vi "TemperatureMeasurePT.vi"(1 "FieldPoint IO Point In":refnum<k21>) -> (0 "Ch1 [K]":dbl)   [LabVIEW 2012]
uses:
  <vilib>/FieldPoint/Polymorphic Read.llb/FP Read (Float -IO).vi
panel:
  in  "?":bool
  # "Temperature Measurement (PT 100)"
  # "(Recommended excitation 1 mA)"
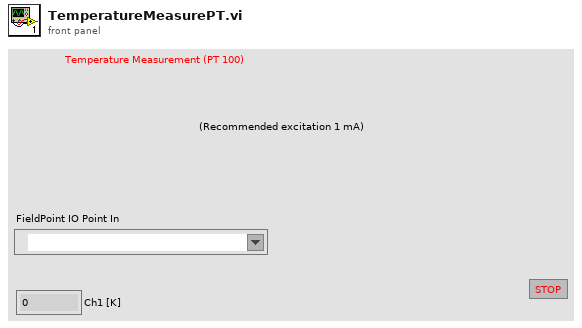
[diagram p1: front panel]
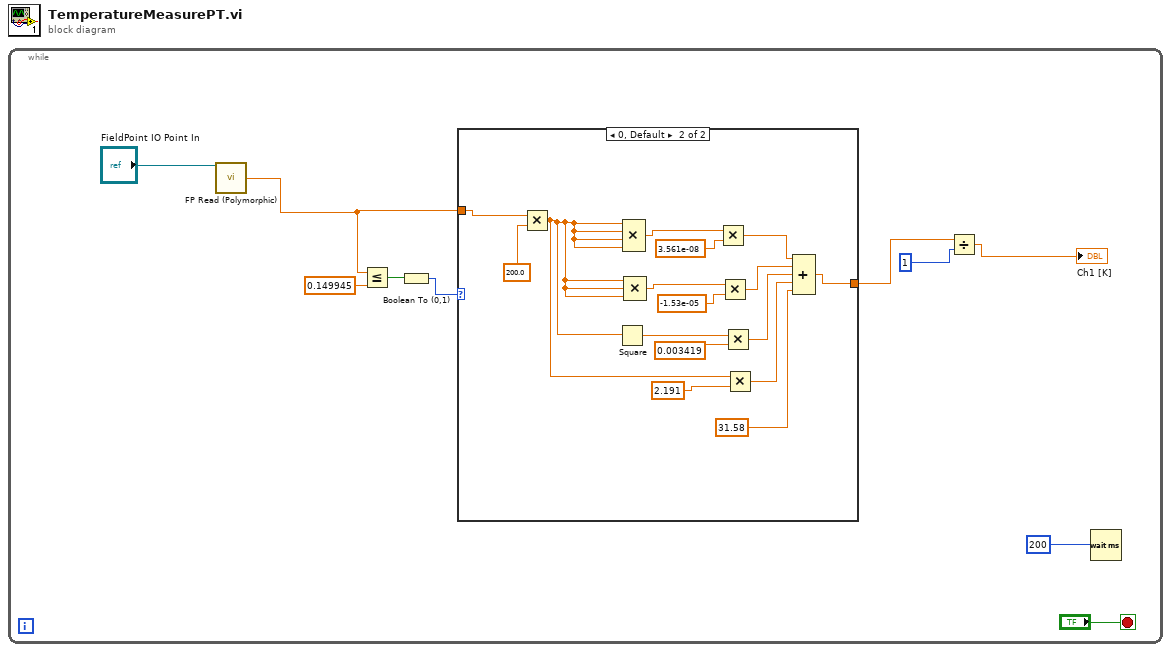
[diagram p0: block diagram]
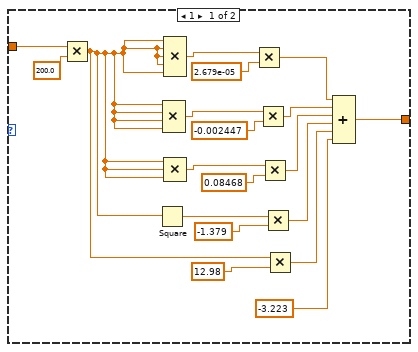
[diagram p2: hidden frame]
diagram:
  n1 = while {
    stop <- "?" stop-if-true
    n2 = call-poly <vilib>:"FP Read (Polymorphic).vi"("FieldPoint IO Point In"="FieldPoint IO Point In") -> ("value"=w4:dbl)  [unwired: 11 in, 3 out]
    n3 = Less Or Equal?(x=w4, y=0.149945) -> (x <= y?=w7:bool)
    n4 = Boolean To (0,1)(Boolean=w7) -> (0, 1=w6:i16)
    n5 = case shown="0, Default" w6 {
      tunnel: w4 -> [w28 w33]
      tunnel: [w17 w31] -> w5
      frame 1 {
        n6 = Multiply(x=w28, y=200.0) -> (x*y=w19:dbl)
        n7 = Square(x=w19) -> (x^2=w21:dbl)
        n8 = Compound Arithmetic op=MULTIPLY(w19, w19, w19, w19) -> (w25:dbl)
        n9 = Compound Arithmetic op=MULTIPLY(w19, w19, w19, w19, w19) -> (w27:dbl)
        n10 = Compound Arithmetic op=MULTIPLY(w19, w19, w19) -> (w23:dbl)
        n11 = Multiply(x=w27, y=2.679e-05) -> (x*y=w16:dbl)
        n12 = Multiply(x=w25, y=-0.002447) -> (x*y=w15:dbl)
        n13 = Multiply(x=w23, y=0.08468) -> (x*y=w14:dbl)
        n14 = Multiply(x=w21, y=-1.379) -> (x*y=w13:dbl)
        n15 = Multiply(x=w19, y=12.98) -> (x*y=w12:dbl)
        n16 = Compound Arithmetic op=ADD(w16, w15, w14, w13, w12, -3.223) -> (w17:dbl)
      }
      frame 0, Default {
        n17 = Multiply(x=w33, y=200.0) -> (x*y=w39:dbl)
        n18 = Square(x=w39) -> (x^2=w41:dbl)
        n19 = Compound Arithmetic op=MULTIPLY(w39, w39, w39, w39) -> (w45:dbl)
        n20 = Compound Arithmetic op=MULTIPLY(w39, w39, w39) -> (w43:dbl)
        n21 = Multiply(x=w45, y=3.561e-08) -> (x*y=w30:dbl)
        n22 = Multiply(x=w43, y=-1.53e-05) -> (x*y=w37:dbl)
        n23 = Multiply(x=w41, y=0.003419) -> (x*y=w36:dbl)
        n24 = Multiply(x=w39, y=2.191) -> (x*y=w35:dbl)
        n25 = Compound Arithmetic op=ADD(w30, w37, w36, w35, 31.58) -> (w31:dbl)
      }
    }
    n26 = Divide(x=w5, y=1) -> (x/y=→"Ch1 [K]":dbl)
    n27 = Wait (ms)(milliseconds to wait=u32 200) -> ()  [unwired: 1 out]
  }
